vi "Zmienne wspoldzielone 0 .vi"() -> ()   [LabVIEW 2020]
panel:
  in  "ON":bool=TRUE
  in  "?":u8(ring) items=["prostokąt", "sinus", "trójkąt"]
  out "PRZEBIEGI":waveform(dbl)(graph)
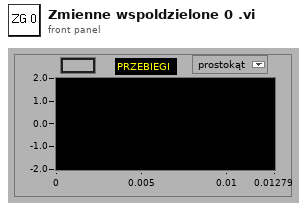
[diagram p1: front panel]
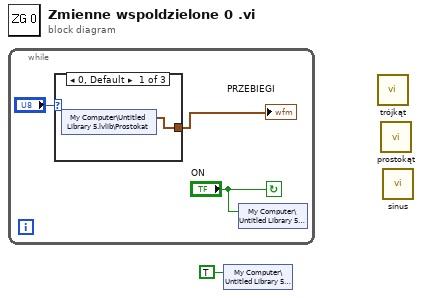
[diagram p0: block diagram]
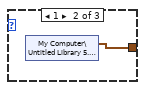
[diagram p2: hidden frame]
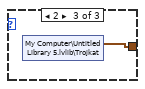
[diagram p3: hidden frame]
diagram:
  n1 = while {
    stop <- "ON" continue-if-true
    n2 = case shown="0, Default" "?" {
      tunnel: [w5 w6 w7] -> w3
      frame 0, Default {
        n3 = shared-variable "My Computer\\Untitled Library 5.lvlib\\Prostokat"() -> (w5:waveform(dbl))  [unwired: 1 in, 1 out]
      }
      frame 1 {
        n4 = shared-variable "My Computer\\Untitled Library 5.lvlib\\Sinus"() -> (w6:waveform(dbl))  [unwired: 1 in, 1 out]
      }
      frame 2 {
        n5 = shared-variable "My Computer\\Untitled Library 5.lvlib\\Trojkat"() -> (w7:waveform(dbl))  [unwired: 1 in, 1 out]
      }
    }
    "PRZEBIEGI" <- w3
    n6 = shared-variable "My Computer\\Untitled Library 5.lvlib\\Stop"("ON") -> ()  [unwired: 1 in, 1 out]
  }
  n7 = shared-variable "My Computer\\Untitled Library 5.lvlib\\Stop"(TRUE ("Stop")) -> ()  [unwired: 1 in, 1 out]
  n8 = call "trójkąt.vi"() -> ()  [unwired: 1 in]
  n9 = call "prostokąt.vi"() -> ()  [unwired: 1 in]
  n10 = call "sinus.vi"() -> ()  [unwired: 1 in]
